vi "CSM - Unregister Status Change.vi"(0 "CSM Name":string, 5 "Source CSM Name (* as Default)":string="*", 7 "Status":string, 9 "Response Message (\"*\" as Default)":string="*", 11 "Error in":errorcluster caption="Error in (no error)") -> (4 "CSM Name(dup)":string, 15 "Error out":errorcluster)   [LabVIEW 2020, in "Communicable State Machine.lvlib"]
doc: "Unregister the notification of other CSM Module's status change.\n\n<b>Inputs:</b>\n - <b>CSM Name</b>: CSM Module name.\n - <b>Source CSM Name</b>: CSM who generates the status. You can use '*' for all modules generated the same <b>Status</b>\n - <b>Status</b>: The status string\n - <b>Error in</b>: Error cluster\n\n<b>Outputs:</b>\n - <b>CSM Name(dup)</b>: return <b>CSM Name</b>\n - <b>Error out</b>: Error cluster"
uses:
  Communicable State Machine.lvlib
  Operation-BroadcastRegistry.ctl
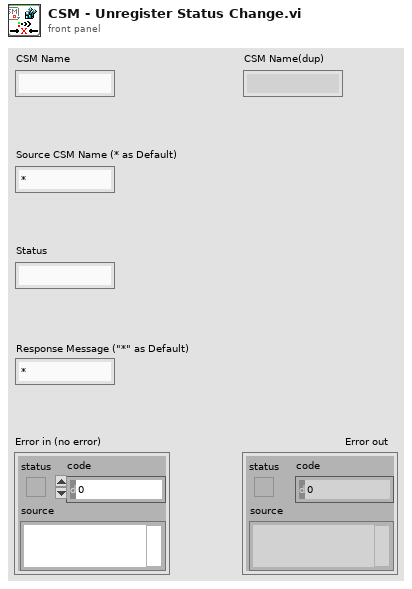
[diagram p1: front panel]
types:
  T1 = typedef "Communicable State Machine.lvlib/Operation-BroadcastRegistry.ctl" = enum16{"Delete Source Module", "Delete Target Module", "Remove Module", "Register", "Unregister", "Check", "List Status", "List Entries"}
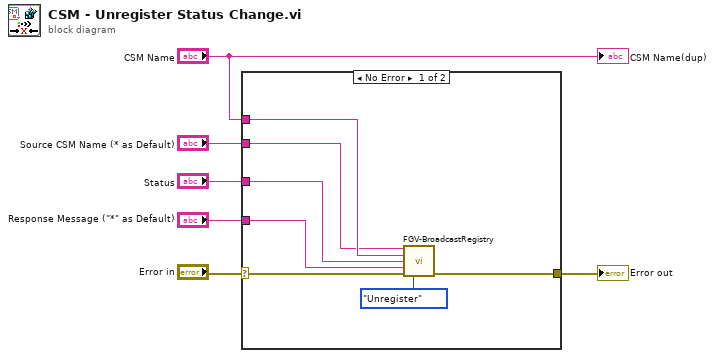
[diagram p0: block diagram]
diagram:
  n1 = case shown="No Error" "Error in" {
    selector: "Error in" -> [w12 w14]
    tunnel: [w11 w14] -> w5
    tunnel: "Response Message (\"*\" as Default)" -> [w10 _]
    tunnel: "Status" -> [w9 _]
    tunnel: "Source CSM Name (* as Default)" -> [w7 _]
    tunnel: "CSM Name" -> [w8 _]
    frame No Error {
      n2 = call "FGV-BroadcastRegistry.vi"("Source"=w7, "Target"=w8, "Status"=w9, "API"=w10, "Error in"=w12, "Operation"=Operation-BroadcastRegistry."Unregister") -> ("Error out"=w11:errorcluster)  [unwired: 8 in, 1 out]
    }
    frame Error {
    }
  }
  "Error out" <- w5
  "CSM Name(dup)" <- "CSM Name"
